vi "Set To Mul.vi"(8 "error in (no error)":errorcluster, 10 "To Mul":dbl, 11 "ByRef Mul in":refnum<class "ByRef Mul.lvclass">) -> (0 "error out":errorcluster, 3 "ByRef Mul out":refnum<class "ByRef Mul.lvclass">)   [LabVIEW 2020, in "ByRef Mul.lvclass"]
uses:
  ByRef Mul.lvclass
  ByRef Mul.lvclass/ByRef Mul.ctl
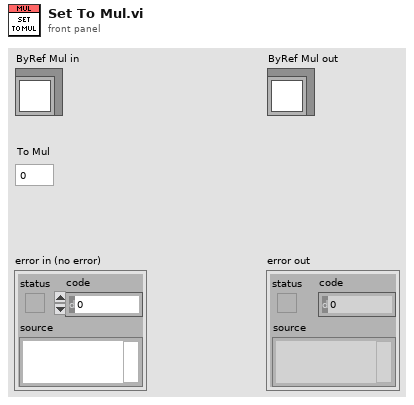
[diagram p1: front panel]
types:
  T1 = typedef "ByRef Mul.lvclass/Ref Data.ctl" = cluster{"To Mul":dbl}
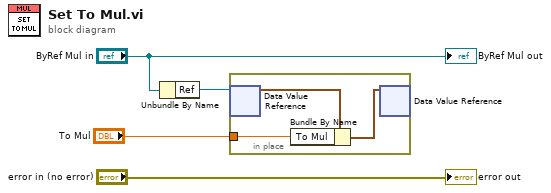
[diagram p0: block diagram]
diagram:
  n1 = Unbundle By Name("ByRef Mul in") -> ("Ref"=w3:refnum<data-value>)
  n2 = in-place {
    in-place-border: "To Mul" -> [w5]
    n3 = in-place-dvr #1(w3) -> (w7:T1)  [unwired: 1 out]
    n4 = Bundle By Name(cluster=w7, "To Mul"=w5) -> (w6:T1)
    n5 = in-place-dvr #1(w6) -> ()  [unwired: 2 out]
  }
  "error out" <- "error in (no error)"
  "ByRef Mul out" <- "ByRef Mul in"
